vi "Tosca-Restore Global AI Properties.vi"(0 "state in":T1) -> (4 "state out":T1)   [LabVIEW 2020]
uses:
  Typedefs/Tosca-AI UI State.ctl
  Typedefs/Tosca-AI Plot Properties.ctl
panel:
  out "error out":errorcluster
  in  "Error In":errorcluster
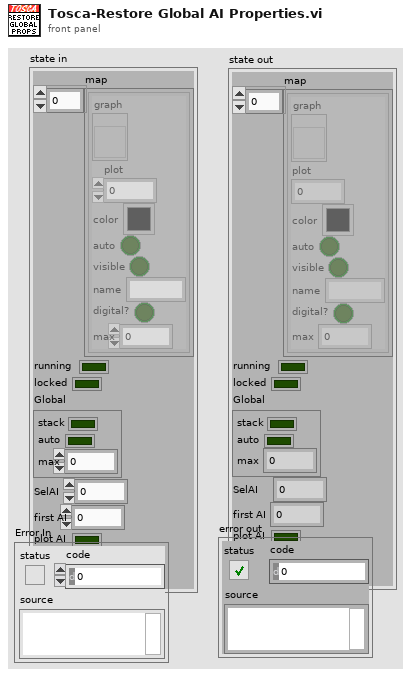
[diagram p1: front panel]
types:
  T1 = typedef "Tosca-AI UI State.ctl" = cluster{"map":T2[], "running":bool, "locked":bool, "Global":cluster{"stack":bool, "auto":bool, "max":dbl}, "SelAI":i32, "first AI":i32, "plot AI":bool, "plot DI":bool, "next":string}
  T2 = typedef "Tosca-AI Plot Properties.ctl" = cluster{"graph":refnum<vi>, "plot":i32, "color":u32, "auto":bool, "visible":bool, "name":string, "digital?":bool, "max":dbl}
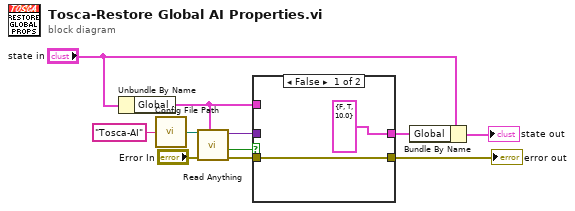
[diagram p0: block diagram]
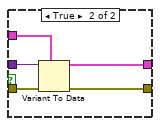
[diagram p2: hidden frame]
diagram:
  n1 = Unbundle By Name("state in") -> ("Global"=w5:cluster{"stack":bool, "auto":bool, "max":dbl})
  n2 = call "Config File Path.vi"("AppName"="Tosca-AI") -> ("Default config file name"=w10:path)
  n3 = call "Read Anything.vi"("Type of Anything"=w5, "Error In"="Error In", "Path (dialog)"=w10) -> ("Error Out"=w9:errorcluster, "Found?"=w8:bool, "Anything"=w6:variant)  [unwired: 6 in]
  n4 = case shown="False" w8 {
    tunnel: w9 -> [w13 w18]
    tunnel: w6 -> [_ w17]
    tunnel: w5 -> [_ w16]
    tunnel: [w13 w15] -> w4
    tunnel: [cluster{"stacked":bool, "auto":bool, "max":dbl} {"stacked"=FALSE, "auto"=TRUE, "max"=10.0} ("Global") w14] -> w2
    frame False {
    }
    frame True {
      n5 = Variant To Data(error in=w18, type=w16, Variant=w17) -> (data=w14:cluster{"stack":bool, "auto":bool, "max":dbl}, error out=w15:errorcluster)
    }
  }
  "error out" <- w4
  n6 = Bundle By Name(cluster="state in", "Global"=w2) -> (→"state out":T1)
